vi "Front Panel Emulator.vi"(10 "Front Panel Emulator Queue in":refnum<queue>, 11 "Device Manager Queue in":refnum<queue>) -> (0 "error out":errorcluster)   [LabVIEW 2026]
uses:
  support/Message Queue/Message Cluster.ctl
  controls/Front Panel Private Data.ctl
  support/Message Queue/Enqueue Message (Single).vi
  <vilib>/Utility/error.llb/Error Cluster From Error Code.vi
  <vilib>/ErrorRing/Error Ring.xnode
  support/Message Queue/Message Queue.lvlib
  support/User Event - Stop/User Event - Stop.lvlib
panel:
  in  "Position":dbl(knob) min=0.0 max=180.0 scale=0.0..180.0
  out "LCD":string
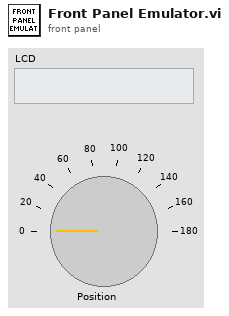
[diagram p1: front panel]
types:
  T1 = typedef "Front Panel Private Data.ctl" = cluster{"Temperature":dbl, "RH":dbl, "Position":dbl}
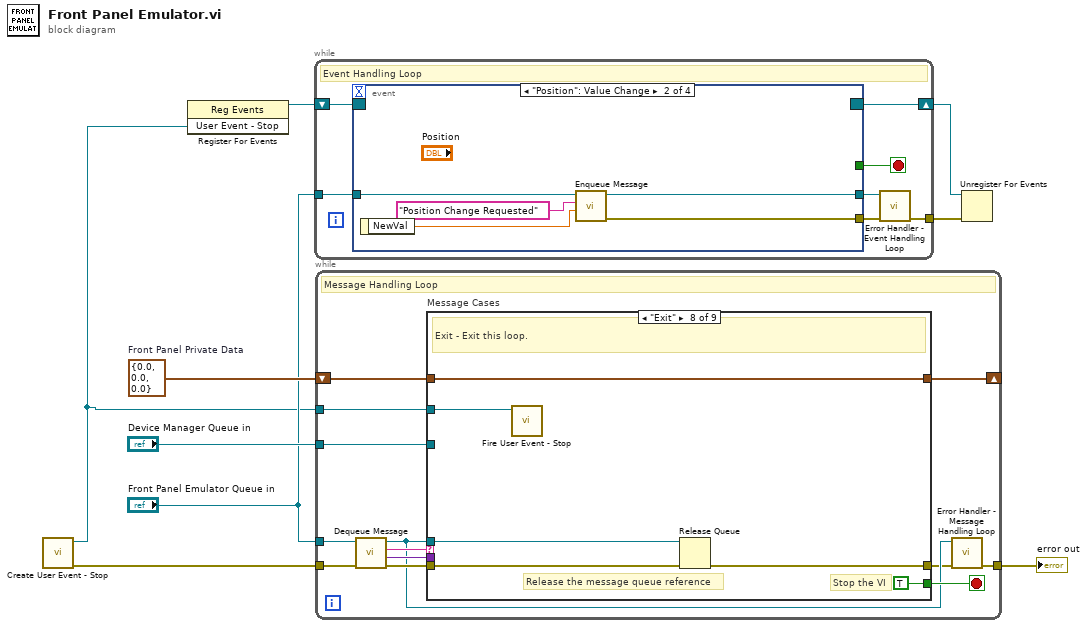
[diagram p0: block diagram]
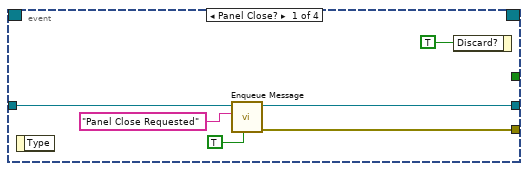
[diagram p2: hidden frame]
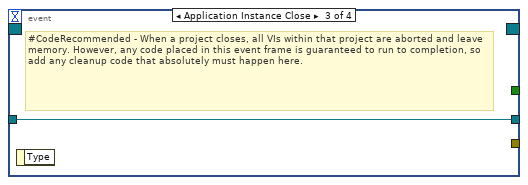
[diagram p3: hidden frame]
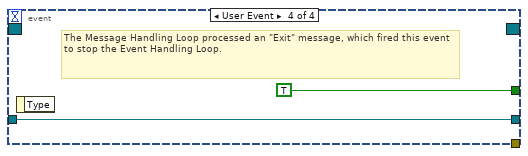
[diagram p4: hidden frame]
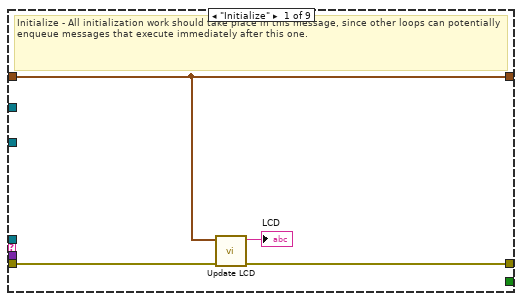
[diagram p5: hidden frame]
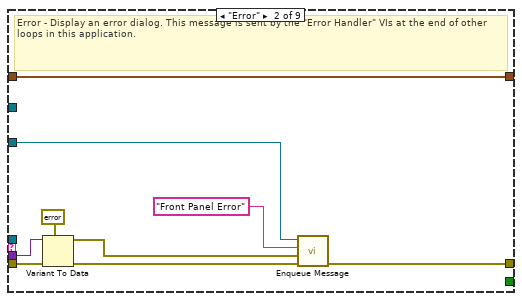
[diagram p6: hidden frame]
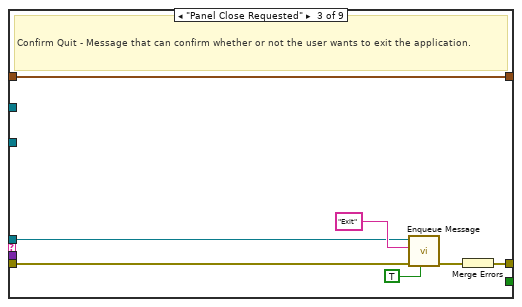
[diagram p7: hidden frame]
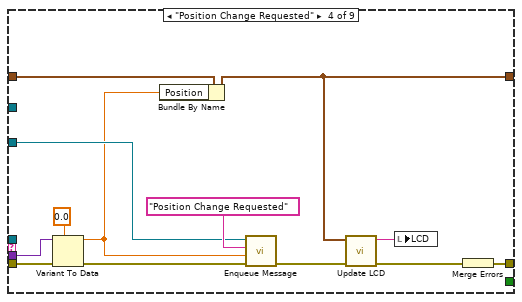
[diagram p8: hidden frame]
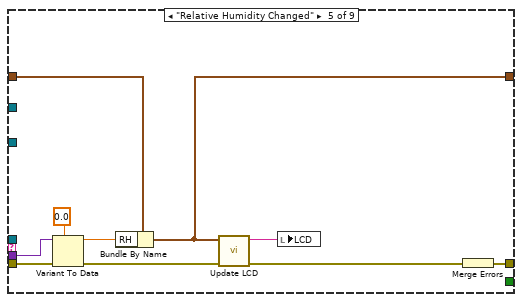
[diagram p9: hidden frame]
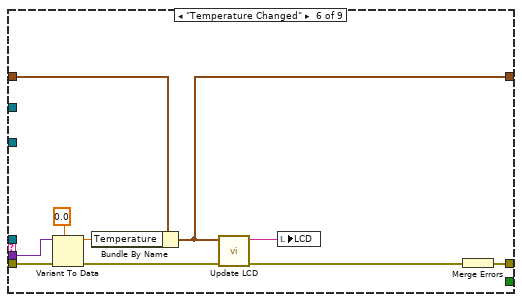
[diagram p10: hidden frame]
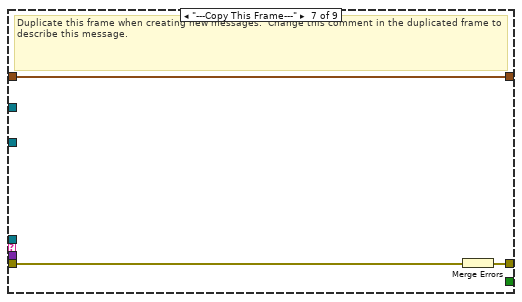
[diagram p11: hidden frame]
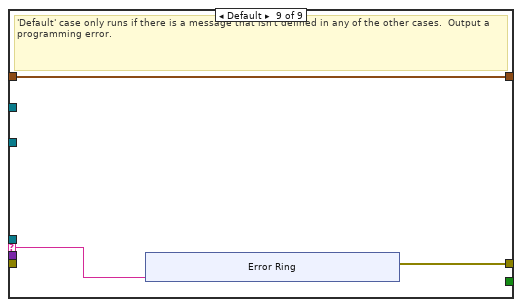
[diagram p12: hidden frame]
diagram:
  w7 = T1 {"Temperature"=0.0, "RH"=0.0, "Position"=0.0}  # Front Panel Private Data
  n1 = call "Create User Event - Stop.vi"() -> ("error out"=w3:errorcluster, "User Event - Stop"=w1:refnum<user-event>)  [unwired: 10 in]
  n2 = register-events(w1) -> (reference out=w4:refnum<event-registration>)  [unwired: 2 in, 1 out]
  n3 = while {
    tunnel: "Front Panel Emulator Queue in" -> [w16]
    shift-right: [w14] -> w6
    shift-left: w4 -> [w15]
    tunnel: [w10] -> w5
    stop <- w12 stop-if-true
    # "Event Handling Loop"
    n4 = event shown="[1] \"Position\": Value Change" {
      selector: w15 -> [_ _ _ _]
      dyn-events: [_ _ _ _] -> w14
      timeout: _ -> [_ _ _ _]
      tunnel: [_ _ _ TRUE ("Discard?")] -> w12
      tunnel: w16 -> [w21 w27 w28 w30]
      tunnel: [w20 w26 _ _] -> w13
      tunnel: [w19 w25 w28 w30] -> w11
      event Panel Close? {
        n5 = event-data() -> ()  [unwired: 1 in, 1 out]
        n6 = call-poly "Enqueue Message.vi"("Priority Message? (F)"=TRUE, "Message"="Panel Close Requested", "Message Queue"=w21) -> ("error out"=w20:errorcluster, "dup Message Queue"=w19:refnum<queue>)  [unwired: 7 in]
        n7 = event-data("Discard?"=TRUE) -> ()  [unwired: 1 in, 1 out]
      }
      event "Position": Value Change {
        n8 = event-data() -> ("NewVal"=w23:dbl)  [unwired: 1 in]
        n9 = call-poly "Enqueue Message.vi"("Message Data"=w23, "Message"="Position Change Requested", "Message Queue"=w27) -> ("error out"=w26:errorcluster, "dup Message Queue"=w25:refnum<queue>)  [unwired: 7 in]
      }
      event Application Instance Close {
        # "#CodeRecommended - When a project closes, all VIs within that project are aborted and leave memory. However, any code placed in this event frame is guaranteed to run to completion, so add any cleanup code that absolutely must happen here."
        n10 = event-data() -> ()  [unwired: 1 in, 1 out]
      }
      event User Event {
        # "The Message Handling Loop processed an \"Exit\" message, which fired this event to stop the Event Handling Loop."
        n11 = event-data() -> ()  [unwired: 1 in, 1 out]
      }
    }
    n12 = call "Error Handler - Event Handling Loop.vi"("error in (no error)"=w13, "Message Queue"=w11) -> ("dup error in"=w10:errorcluster)  [unwired: 8 in, 1 out]
  }
  n13 = while {
    tunnel: "Front Panel Emulator Queue in" -> [w36]
    shift-right: [w42] -> _
    shift-left: w7 -> [w43]
    tunnel: w3 -> [w40]
    tunnel: [w34] -> w9
    tunnel: "Device Manager Queue in" -> [w32]
    tunnel: w1 -> [w31]
    stop <- w41 stop-if-true
    # "Message Handling Loop"
    n14 = call "Dequeue Message.vi"("error in (no error)"=w40, "Message Queue"=w36) -> ("error out"=w39:errorcluster, "Message Data"=w37:variant, "Message"=w38:string, "dup Message Queue"=w35:refnum<queue>)  [unwired: 6 in]
    n15 = case "Message Cases" shown="\"Exit\"" w38 {
      selector: w38 -> [_ _ _ _ _ _ _ _ w106]
      tunnel: w35 -> [_ _ w57 _ _ _ _ w105 _]
      tunnel: w39 -> [w45 w56 w63 w69 w82 w92 w99 w101 _]
      tunnel: [w46 w49 w61 w75 w85 w95 w97 w102 w107] -> w33
      tunnel: w43 -> [w47 w55 w62 w76 w86 w96 w98 w104 w108]
      tunnel: [w47 w55 w62 w67 w78 w88 w98 w104 w108] -> w42
      tunnel: [_ _ _ _ _ _ _ TRUE _] -> w41
      tunnel: w37 -> [_ w54 _ w72 w83 w93 _ _ _]
      tunnel: w32 -> [_ w48 _ w71 _ _ _ _ _]
      tunnel: w31 -> [_ _ _ _ _ _ _ w100 _]
      frame "Initialize" {
        # "Initialize - All initialization work should take place in this message, since other loops can potentially enqueue messages that execute immediately after this one."
        n16 = call "Update LCD.vi"("error in"=w45, "Front Panel Private Data in"=w47) -> ("error out"=w46:errorcluster, "LCD"=→"LCD":string)  [unwired: 8 in]
      }
      frame "Error" {
        # "Error - Display an error dialog. This message is sent by the \"Error Handler\" VIs at the end of other loops in this application."
        n17 = Variant To Data(error in=w56, type=errorcluster {"status"=FALSE, "code"=0, "source"=""} ("error constant"), Variant=w54) -> (data=w51:errorcluster, error out=w50:errorcluster)
        n18 = call-poly "Enqueue Message.vi"("error in (no error)"=w50, "Message Data"=w51, "Message"="Front Panel Error", "Message Queue"=w48) -> ("error out"=w49:errorcluster)  [unwired: 6 in, 1 out]
      }
      frame "Panel Close Requested" {
        # "Confirm Quit - Message that can confirm whether or not the user wants to exit the application."
        n19 = call-poly "Enqueue Message.vi"("Priority Message? (F)"=TRUE, "error in (no error)"=w63, "Message"="Exit", "Message Queue"=w57) -> ("error out"=w60:errorcluster)  [unwired: 6 in, 1 out]
        n20 = Merge Errors(w60) -> (w61:errorcluster)
      }
      frame "Position Change Requested" {
        n21 = Variant To Data(error in=w69, type=0.0 ("Position"), Variant=w72) -> (data=w68:dbl, error out=w70:errorcluster)
        n22 = Bundle By Name(cluster=w76, "Position"=w68) -> (w67:T1)
        n23 = call-poly "Enqueue Message.vi"("error in (no error)"=w70, "Message Data"=w68, "Message"="Position Change Requested", "Message Queue"=w71) -> ("error out"=w66:errorcluster)  [unwired: 6 in, 1 out]
        n24 = call "Update LCD.vi"("error in"=w66, "Front Panel Private Data in"=w67) -> ("error out"=w65:errorcluster, "LCD"=w64:string)  [unwired: 8 in]
        n25 = local write "LCD"(w64) -> ()
        n26 = Merge Errors(w65) -> (w75:errorcluster)
      }
      frame "Relative Humidity Changed" {
        n27 = Variant To Data(error in=w82, type=0.0 ("Position"), Variant=w83) -> (data=w81:dbl, error out=w80:errorcluster)
        n28 = Bundle By Name(cluster=w86, "RH"=w81) -> (w78:T1)
        n29 = call "Update LCD.vi"("error in"=w80, "Front Panel Private Data in"=w78) -> ("error out"=w79:errorcluster, "LCD"=w77:string)  [unwired: 8 in]
        n30 = local write "LCD"(w77) -> ()
        n31 = Merge Errors(w79) -> (w85:errorcluster)
      }
      frame "Temperature Changed" {
        n32 = Variant To Data(error in=w92, type=0.0 ("Position"), Variant=w93) -> (data=w91:dbl, error out=w90:errorcluster)
        n33 = Bundle By Name(cluster=w96, "Temperature"=w91) -> (w88:T1)
        n34 = call "Update LCD.vi"("error in"=w90, "Front Panel Private Data in"=w88) -> ("error out"=w89:errorcluster, "LCD"=w87:string)  [unwired: 8 in]
        n35 = local write "LCD"(w87) -> ()
        n36 = Merge Errors(w89) -> (w95:errorcluster)
      }
      frame "---Copy This Frame---" {
        # "Duplicate this frame when creating new messages.  Change this comment in the duplicated frame to describe this message."
        n37 = Merge Errors(w99) -> (w97:errorcluster)
      }
      frame "Exit" {
        # "Stop the VI"
        # "Release the message queue reference"
        # "Exit - Exit this loop."
        n38 = call "Fire User Event - Stop.vi"("User Event - Stop"=w100) -> ()  [unwired: 10 in, 1 out]
        n39 = Release Queue(queue=w105, error in (no error)=w101) -> (error out=w102:errorcluster)  [unwired: 1 in, 2 out]
      }
      frame Default {
        # "'Default' case only runs if there is a message that isn't defined in any of the other cases.  Output a programming error."
        n40 = xnode "Error Ring"("parameter 0"=w106) -> ("error out"=w107:errorcluster)
      }
    }
    n41 = call "Error Handler - Message Handling Loop.vi"("error in (no error)"=w33, "Message Queue"=w35) -> ("dup error in"=w34:errorcluster)  [unwired: 8 in, 1 out]
  }
  "error out" <- w9
  n42 = Unregister For Events(event registration refnum=w6, error in=w5) -> ()  [unwired: 1 out]
